vi "Table, Copy Column Colors.vi"(4 "dst col (0)":i32, 5 "src col (0)":i32, 6 "dst row (0)":i32, 7 "src row (0)":i32, 8 "error in":errorcluster, 9 "n rows (1)":i32=1, 10 "Tbl Refnum Dst":refnum<vi>, 11 "Tbl Refnum Src":refnum<vi>) -> (0 "error out":errorcluster, 2 "Tbl Refnum Dst out":refnum<vi>, 3 "Tbl Refnum Src out":refnum<vi>)   [LabVIEW 2010]
doc: "This function copies cell background color attributes fom a source table column to a destination table column."
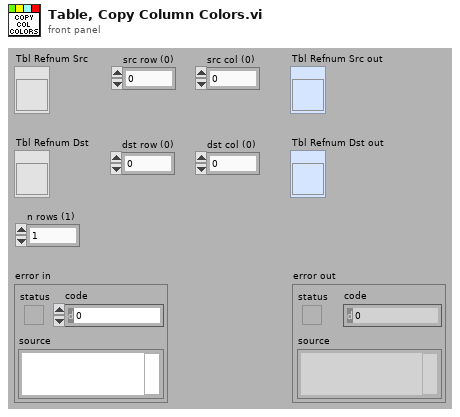
[diagram p1: front panel]
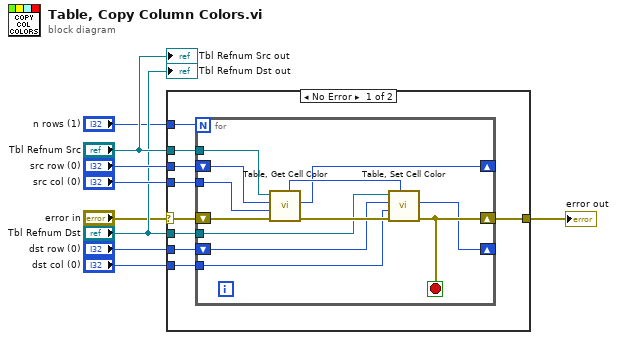
[diagram p0: block diagram]
diagram:
  n1 = case shown="No Error" "error in" {
    selector: "error in" -> [w11 w31]
    tunnel: [w18 w31] -> w9
    tunnel: "dst row (0)" -> [w17 _]
    tunnel: "dst col (0)" -> [w16 _]
    tunnel: "src col (0)" -> [w15 _]
    tunnel: "src row (0)" -> [w14 _]
    tunnel: "Tbl Refnum Src" -> [w13 _]
    tunnel: "Tbl Refnum Dst" -> [w12 _]
    tunnel: "n rows (1)" -> [w10 _]
    frame No Error {
      n2 = for {
        N: w10 -> [_]
        shift-right: [w25] -> w18
        shift-left: w11 -> [w28]
        tunnel: w13 -> [w27]
        tunnel: w12 -> [w26]
        shift-right: [w23] -> _
        shift-left: w14 -> [w24]
        shift-right: [w19] -> _
        shift-left: w17 -> [w20]
        tunnel: w16 -> [w21]
        tunnel: w15 -> [w22]
        stop <- w25 stop-if-true
        n3 = call "Table, Get Cell Color.vi"("error in"=w28, "col (0)"=w22, "row (0)"=w24, "Tbl Refnum"=w27) -> ("error out"=w30:errorcluster, "row+1"=w23:i32, "BGColor"=w29:u32)  [unwired: 3 in, 2 out]
        n4 = call "Table, Set Cell Color.vi"("BGColor Enabled"=w29, "error in"=w30, "col (0)"=w21, "row (0)"=w20, "Tbl Refnum"=w26) -> ("error out"=w25:errorcluster, "row+1"=w19:i32)  [unwired: 2 in, 2 out]
      }
    }
    frame Error {
    }
  }
  "error out" <- w9
  "Tbl Refnum Src out" <- "Tbl Refnum Src"
  "Tbl Refnum Dst out" <- "Tbl Refnum Dst"
